vi "Match Numeric Array to String Array Size.vi"(7 "String Array":string[](array[string]), 10 "Max Size":i32, 11 "Numeric Array in":i32[](array[numeric])) -> (2 "Exceeded Max Size":bool, 3 "Numeric Array out":i32[](array[numeric]))   [LabVIEW 2015, in "NI_AWS_SQS.lvclass"]
uses:
  NI_AWS_SQS.lvclass
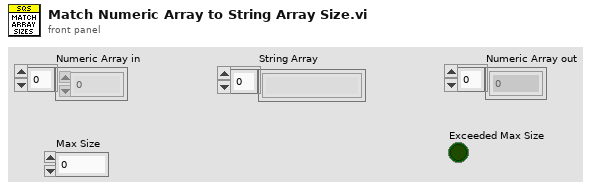
[diagram p1: front panel]
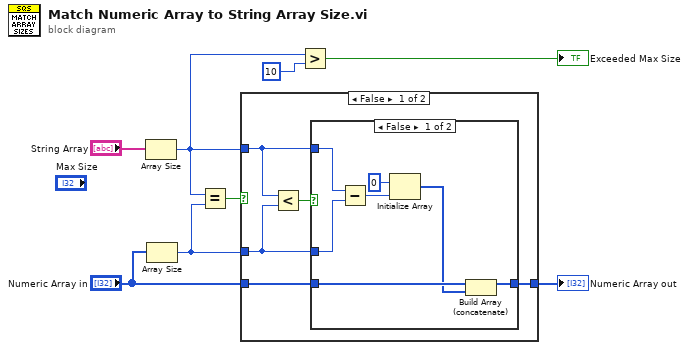
[diagram p0: block diagram]
diagram:
  n1 = Array Size(array="String Array") -> (size(s)=w3:i32)
  n2 = Array Size(array="Numeric Array in") -> (size(s)=w4:i32)
  n3 = Equal?(x=w3, y=w4) -> (x = y?=w7:bool)
  n4 = case shown="False" w7 {
    tunnel: "Numeric Array in" -> [w13 w22]
    tunnel: [w11 w22] -> w5
    tunnel: w3 -> [w9 _]
    tunnel: w4 -> [w10 _]
    frame False {
      n5 = Less?(x=w9, y=w10) -> (x < y?=w12:bool)
      n6 = case shown="False" w12 {
        tunnel: w13 -> [w16 w21]
        tunnel: [w15 w21] -> w11
        tunnel: w10 -> [w19 _]
        tunnel: w9 -> [w20 _]
        frame False {
          n7 = Subtract(x=w20, y=w19) -> (x-y=w18:i32)
          n8 = Initialize Array(0, w18) -> (w14:i32[])
          n9 = Build Array (concatenate)(w16, w14) -> (w15:i32[])
        }
        frame True {
        }
      }
    }
    frame True {
    }
  }
  "Numeric Array out" <- w5
  n10 = Greater?(x=w3, y=10) -> (0:→"Exceeded Max Size":bool)
